vi "Execute Turn.vi"(8 "error in":errorcluster, 11 "Reversi in":refnum<class "Reversi.lvclass">) -> (0 "error out":errorcluster, 3 "Reversi out":refnum<class "Reversi.lvclass">)   [LabVIEW 2020, in "Reversi.lvlib" / "Reversi.lvclass"]
uses:
  Reversi.lvclass
  Reversi.lvclass/Reversi.ctl
  Space Cluster.ctl
  Space Coordinates.ctl
  Space Ring.ctl
  Turn Enum.ctl
  Player/Player.lvclass
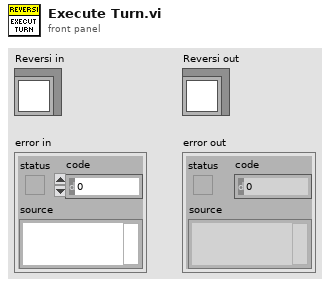
[diagram p1: front panel]
types:
  T1 = typedef "Reversi.lvlib/Reversi.lvclass/Turn Enum.ctl" = enum16{"Black", "White"}
  T2 = typedef "Reversi.lvlib/Reversi.lvclass/Space Ring.ctl" = u16
  T3 = typedef "Reversi.lvlib/Reversi.lvclass/Space Cluster.ctl" = cluster{"Coordinates":T4, "Ring":T2}
  T4 = typedef "Reversi.lvlib/Reversi.lvclass/Space Coordinates.ctl" = cluster{"Row":i32, "Column":i32}
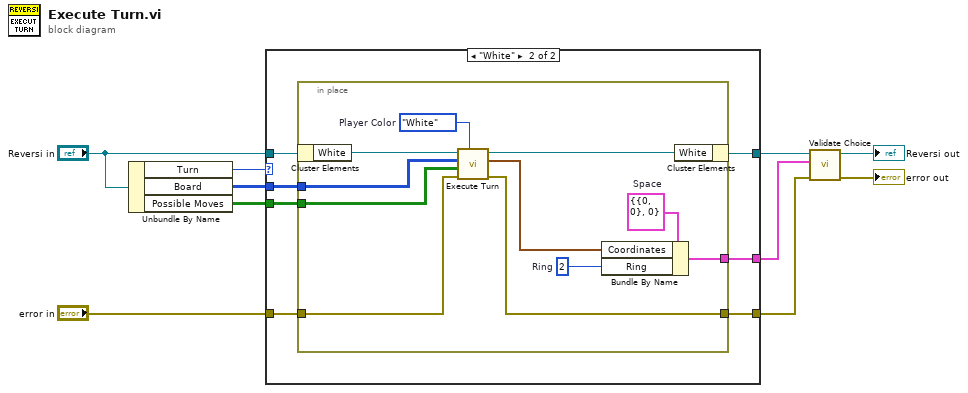
[diagram p0: block diagram]
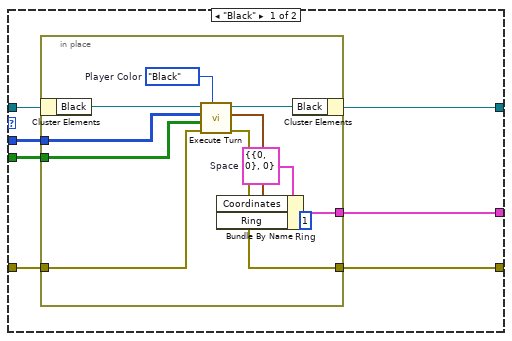
[diagram p2: hidden frame]
diagram:
  n1 = Unbundle By Name("Reversi in") -> ("Turn"=w4:T1, "Board"=w6:T2[][], "Possible Moves"=w5:bool[][])
  n2 = case shown="\"White\"" w4 {
    tunnel: "Reversi in" -> [w15 w33]
    tunnel: w6 -> [w14 w32]
    tunnel: w5 -> [w13 w31]
    tunnel: "error in" -> [w17 w35]
    tunnel: [w12 w30] -> w3
    tunnel: [w11 w29] -> w2
    tunnel: [w16 w34] -> w9
    frame "Black" {
      n3 = in-place {
        in-place-border: w14 -> [w24]
        in-place-border: w13 -> [w23]
        in-place-border: w17 -> [w28]
        in-place-border: [w27] -> w16
        in-place-border: [w19] -> w11
        w18 = Turn_Enum."Black"  # Player Color
        w20 = T2 1  # Ring
        w22 = T3 {"Coordinates"={"Row"=0, "Column"=0}, "Ring"=0}  # Space
        n4 = in-place-cluster #1(w15) -> ("Black"=w26:refnum<class "Player.lvclass">)
        n5 = call-dynamic "Execute Turn.vi"("Player Color"=w18, "error in"=w28, "Possible Moves"=w23, "Board"=w24, "Player in"=w26) -> ("error out"=w27:errorcluster, "Choice Coordinates"=w21:T4, "Player out"=w25:refnum<class "Player.lvclass">)  [unwired: 4 in]
        n6 = Bundle By Name(cluster=w22, "Coordinates"=w21, "Ring"=w20) -> (w19:T3)
        n7 = in-place-cluster #1("Black"=w25) -> (w12:refnum<class "Reversi.lvclass">)
      }
    }
    frame "White" {
      n8 = in-place {
        in-place-border: w32 -> [w42]
        in-place-border: w31 -> [w37]
        in-place-border: w35 -> [w46]
        in-place-border: [w45] -> w34
        in-place-border: [w39] -> w29
        w38 = Turn_Enum."White"  # Player Color
        w40 = T2 2  # Ring
        w41 = T3 {"Coordinates"={"Row"=0, "Column"=0}, "Ring"=0}  # Space
        n9 = in-place-cluster #2(w33) -> ("White"=w44:refnum<class "Player.lvclass">)
        n10 = call-dynamic "Execute Turn.vi"("Player Color"=w38, "error in"=w46, "Possible Moves"=w37, "Board"=w42, "Player in"=w44) -> ("error out"=w45:errorcluster, "Choice Coordinates"=w36:T4, "Player out"=w43:refnum<class "Player.lvclass">)  [unwired: 4 in]
        n11 = Bundle By Name(cluster=w41, "Coordinates"=w36, "Ring"=w40) -> (w39:T3)
        n12 = in-place-cluster #2("White"=w43) -> (w30:refnum<class "Reversi.lvclass">)
      }
    }
  }
  n13 = call "Validate Choice.vi"("error in (no error)"=w9, "Choice"=w2, "Reversi in"=w3) -> ("error out"=→"error out":errorcluster, "Reversi out"=→"Reversi out":refnum<class "Reversi.lvclass">)  [unwired: 7 in]
